vi "Configure Channel (Voltage Range).vi"(7 "Voltage Range (5V)":dbl=5.0, 8 "error in (no error)":errorcluster, 9 "Probe Factor ( 1:1)":i32(ring)=1 items=["1:1"=1, "10:1"=10], 10 "Channel (1: Channel 1)":i32(ring)=1 items=["Channel 1"=1, "Channel 2"=2], 11 "VISA resource name":refnum<visa-resource-name>) -> (0 "error out":errorcluster, 3 "VISA resource name out":refnum<visa-resource-name>)   [LabVIEW 2024, in "Agilent 532XX Series.lvlib"]
doc: "Selects the probe factor (1:1 or 10:1) for the input channel, and specifies voltage range according to the probe factor."
uses:
  Agilent 532XX Series.lvlib
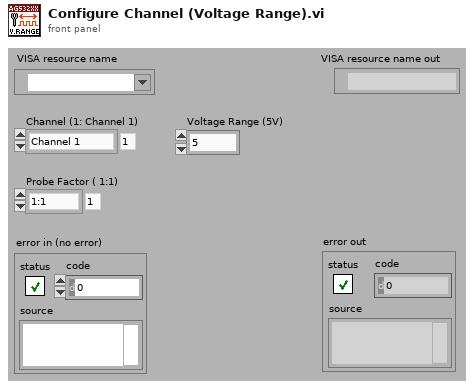
[diagram p1: front panel]
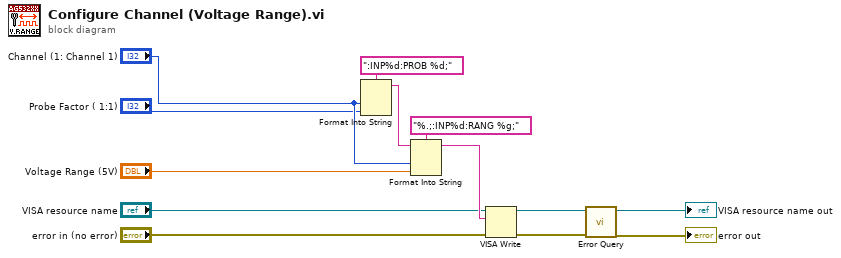
[diagram p0: block diagram]
diagram:
  n1 = Format Into String(format string=":INP%d:PROB %d;", "Channel (1: Channel 1)", "Probe Factor ( 1:1)") -> (resulting string=w10:string)  [unwired: 2 in, 1 out]
  n2 = Format Into String(format string="%.;:INP%d:RANG %g;", initial string=w10, "Channel (1: Channel 1)", "Voltage Range (5V)") -> (resulting string=w7:string)  [unwired: 1 in, 1 out]
  n3 = VISA Write(VISA resource name="VISA resource name", write buffer=w7, error in (no error)="error in (no error)") -> (VISA resource name out=w4:refnum<visa-resource-name>, error out=w3:errorcluster)  [unwired: 1 out]
  n4 = call "Error Query.vi"("error in (no error)"=w3, "VISA resource name"=w4) -> ("error out"=→"error out":errorcluster, "VISA resource name out"=→"VISA resource name out":refnum<visa-resource-name>)  [unwired: 8 out]
